vi "mod0 sub.vi"(0 "Array":i32[][](array[numeric])) -> (1 "Array 2":i32[][](array[numeric]), 2 "new picture":picture)   [LabVIEW 2010]
panel:
  in  "GC-Sequenz ändern":bool
  out "?":i32[](array[numeric])
  in  "?":i32[](array[numeric])
  in  "multipos":bool
  in  "pump2 ändern":bool
  in  "pump1 ändern":bool
  out "mod0 pump2":bool
  out "mod0 pump1":bool
  in  "mod0 zurück":bool
  # "GC-Sequenz:\n\n1=Luftprobe\n2=Blank\n3=Blank-to-Pump\n4=Standard1\n5=Standard2\n6=Standard3"
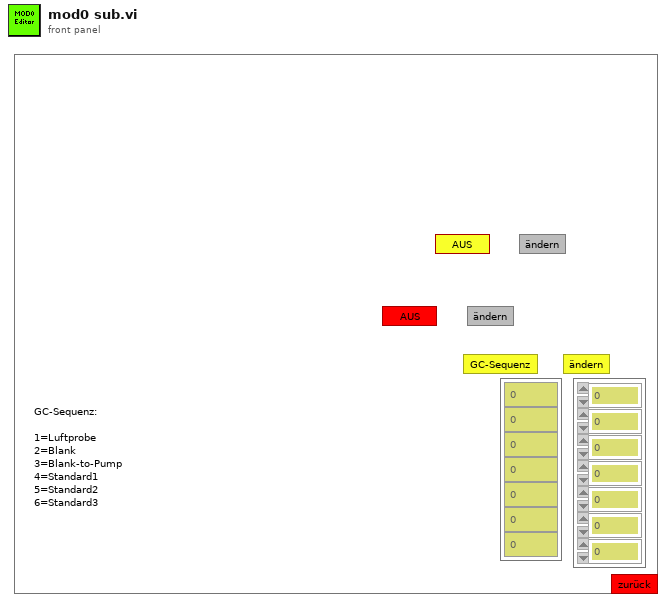
[diagram p1: front panel]
types:
  T1 = typedef "imagedata.ctl" = cluster{"image type":i32, "image depth":i32, "image":u8[], "mask":u8[], "colors":u32[], "Rectangle":cluster{"left":i16, "top":i16, "right":i16, "bottom":i16}}
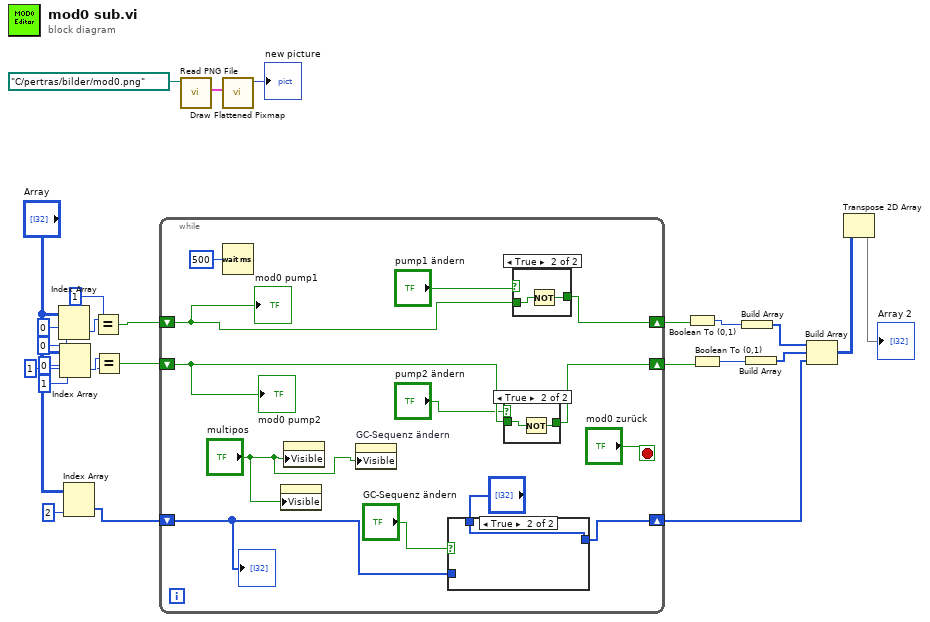
[diagram p0: block diagram]
diagram:
  n1 = Index Array(array="Array", index (row)=0 ("Index (Zeile)"), index (col)=0 ("Deaktivierter Index (Spalte)")) -> (element=w19:i32)
  n2 = Index Array(array="Array", index (row)=0 ("Index (Zeile)"), index (col)=1 ("Deaktivierter Index (Spalte)")) -> (element=w14:i32)
  n3 = Index Array(array="Array", index (col)=2 ("Deaktivierter Index (Spalte)")) -> (element=w10:i32[])  [unwired: 1 in]
  n4 = Equal?(x=w19, y=1) -> (x = y?=w17:bool)
  n5 = Equal?(x=w14, y=1) -> (x = y?=w12:bool)
  n6 = while {
    shift-right: [w31] -> w9
    shift-left: w17 -> [w37]
    shift-right: [w32] -> w8
    shift-left: w12 -> [w36]
    shift-right: [w29] -> w3
    shift-left: w10 -> [w27]
    stop <- "mod0 zurück" stop-if-true
    n7 = Wait (ms)(milliseconds to wait=u32 500 ("Zu wartende ms")) -> ()  [unwired: 1 out]
    n8 = property class="Arr (strikt)"("Visible"="multipos") -> ()  [unwired: 2 in, 2 out]
    n9 = property class="Arr (strikt)"("Visible"="multipos") -> ()  [unwired: 2 in, 2 out]
    n10 = property on="GC-Sequenz ändern" class="Bool."("Visible"="multipos") -> ()  [unwired: 2 in, 2 out]
    n11 = case shown="True" "GC-Sequenz ändern" {
      tunnel: "?" -> [_ w40]
      tunnel: [w39 w40] -> w29
      tunnel: w27 -> [w39 _]
      frame False {
      }
      frame True {
      }
    }
    n12 = case shown="True" "pump2 ändern" {
      tunnel: w36 -> [w41 w43]
      tunnel: [w41 w42] -> w32
      frame False {
      }
      frame True {
        n13 = Not(x=w43) -> (.not. x?=w42:bool)
      }
    }
    n14 = case shown="True" "pump1 ändern" {
      tunnel: w37 -> [w44 w46]
      tunnel: [w44 w45] -> w31
      frame False {
      }
      frame True {
        n15 = Not(x=w46) -> (.not. x?=w45:bool)
      }
    }
    "mod0 pump1" <- w37
    "mod0 pump2" <- w36
    "?" <- w27
  }
  n16 = call <vilib>:"Read PNG File.vi"("path to PNG file"=path "C:/pertras/bilder/mod0.png") -> ("image data"=w23:T1)  [unwired: 8 in, 2 out]
  n17 = call <vilib>:"Draw Flattened Pixmap.vi"("image data"=w23) -> ("new picture"=→"new picture":picture)  [unwired: 8 in]
  n18 = Boolean To (0,1)(Boolean=w9) -> (0, 1=w7:i16)
  n19 = Boolean To (0,1)(Boolean=w8) -> (0, 1=w6:i16)
  n20 = Build Array(w7) -> (w5:i16[])
  n21 = Build Array(w6) -> (w4:i16[])
  n22 = Build Array(w5, w4, w3) -> (w2:i32[][])
  n23 = Transpose 2D Array(2D array=w2) -> (transposed array=→"Array 2":i32[][])
